vi "convert Celsius to Kelvin.vi"(5 "T [C]":dbl[](array[numeric])) -> (6 "T [K]":dbl[](array[numeric]))   [LabVIEW 2010, in "util.lvlib"]
uses:
  util.lvlib
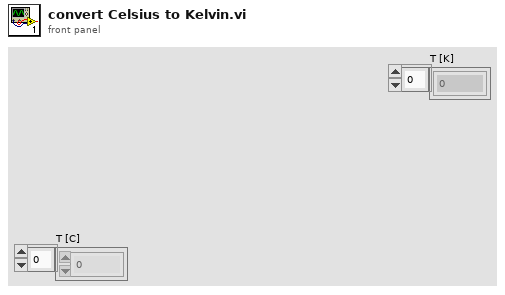
[diagram p1: front panel]
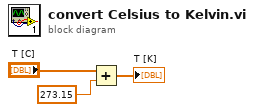
[diagram p0: block diagram]
diagram:
  n1 = Add(x="T [C]", y=273.15) -> (x+y=→"T [K]":dbl[])
